vi "__uintDivide.vi"(8 "Base (decimal)":T1=10 items=["Binary"=2, "Octal"=8, "Decimal"=10, "Hexadecimal"=16, "Hexatrigesimal"=36, "ASCII"=64], 10 "Uint2 in":u8[](array[numeric]), 11 "Uint1 in":u8[](array[numeric])) -> (0 "Timing division":u32, 2 "floor(Uint1 / Uint1)":u8[](array[numeric]), 3 "Uint1 mod Uint2":u8[](array[numeric]))   [LabVIEW 2011, in "UintClass.lvclass"]
uses:
  UintClass.lvclass
  enumBase.ctl
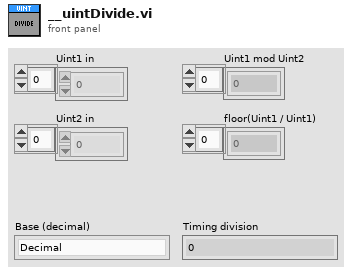
[diagram p1: front panel]
types:
  T1 = typedef "UintClass.lvclass/enumBase.ctl" = u16
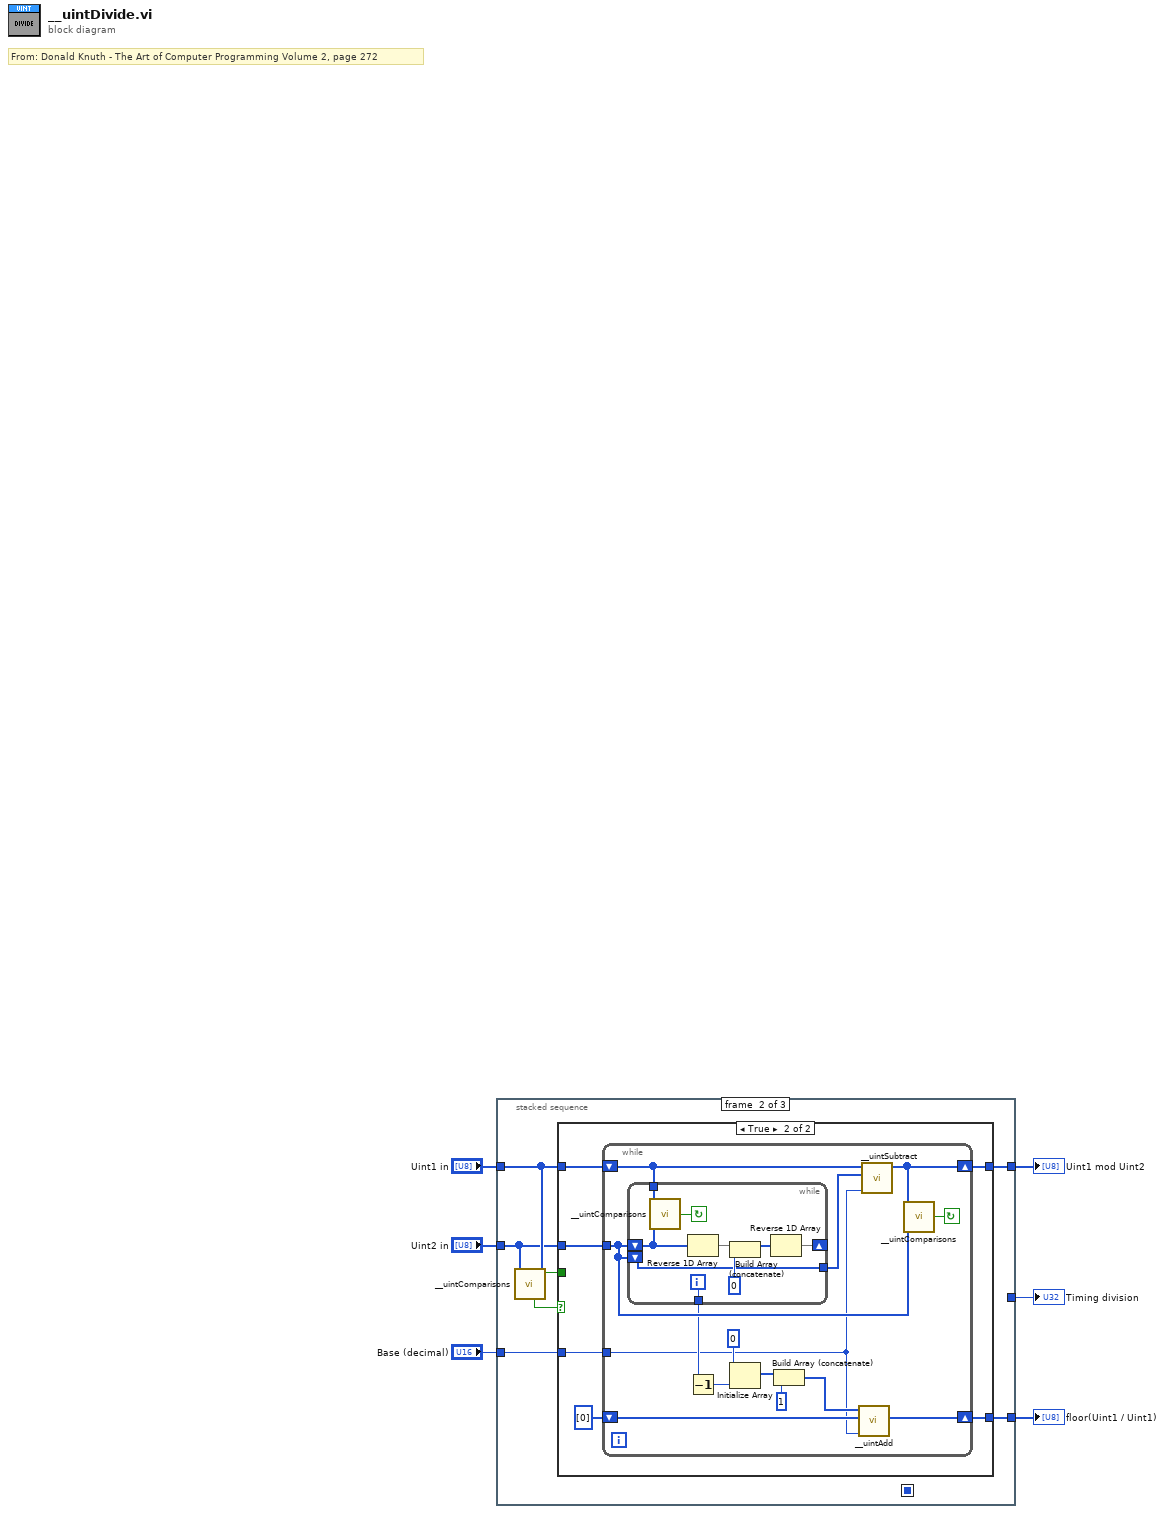
[diagram p0: block diagram]
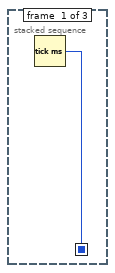
[diagram p2: hidden frame]
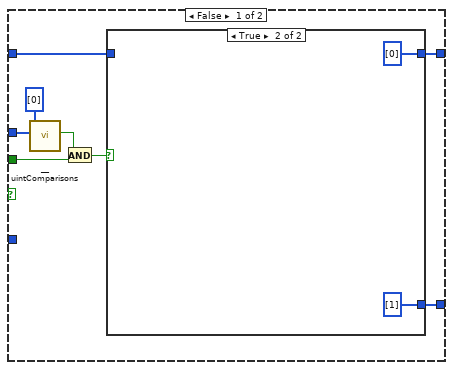
[diagram p3: hidden frame]
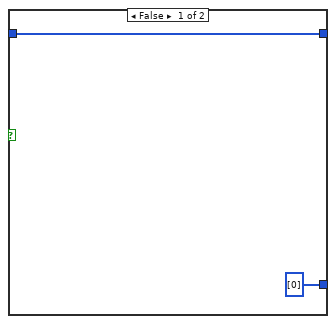
[diagram p4: hidden frame]
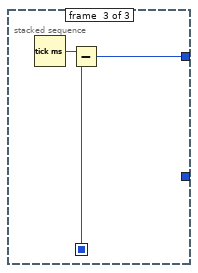
[diagram p5: hidden frame]
diagram:
  # "From: Donald Knuth - The Art of Computer Programming Volume 2, page 272"
  n1 = stacked-sequence {
    seq-local: [w7 _ _] -> [_ _ w57]
    tunnel: "Uint2 in" -> [_ w12 _]
    tunnel: "Uint1 in" -> [_ w13 _]
    tunnel: "Base (decimal)" -> [_ w14 _]
    tunnel: [_ w10 _] -> w4
    tunnel: [_ w11 _] -> w3
    tunnel: [_ _ w56] -> w1
    frame #0 {
      n2 = Tick Count (ms)() -> (millisecond timer value=w7:u32)
    }
    frame #1 {
      n3 = call "__uintComparisons.vi"("Uint2 in"=w12, "Uint1 in"=w13) -> ("Uint1 = Uint2"=w8:bool, "Uint1 > Uint2"=w9:bool)  [unwired: 3 in, 5 out]
      n4 = case shown="True" w9 {
        tunnel: w14 -> [_ w30]
        tunnel: w13 -> [w22 w32]
        tunnel: w12 -> [w19 w31]
        tunnel: [w21 w28] -> w11
        tunnel: [w20 w27] -> w10
        tunnel: w8 -> [w17 _]
        frame False {
          n5 = call "__uintComparisons.vi"("Uint2 in"=w19, "Uint1 in"=u8[] [0]) -> ("Uint1 != Uint2"=w15:bool)  [unwired: 3 in, 6 out]
          n6 = And(x=w15, y=w17) -> (x .and. y?=w16:bool)
          n7 = case shown="True" w16 {
            tunnel: w22 -> [w24 _]
            tunnel: [w24 u8[] [0] ("Uint2 in")] -> w21
            tunnel: [u8[] [0] ("Uint2 in") u8[] [1] ("Uint2 in")] -> w20
            frame False {
            }
            frame True {
            }
          }
        }
        frame True {
          n8 = while {
            tunnel: w31 -> [w44]
            tunnel: w30 -> [w34]
            shift-right: [w35] -> w28
            shift-left: w32 -> [w46]
            shift-right: [w36] -> w27
            shift-left: u8[] [0] ("Uint2 in") -> [w37]
            stop <- w33 continue-if-true
            n9 = while {
              tunnel: w46 -> [w55]
              shift-right: [w49] -> _
              shift-left: w44 -> [w53]
              shift-left: w44 -> [w48]
              tunnel: [w48] -> w45
              tunnel: [w47] -> w39
              i -> [w47]
              stop <- w54 continue-if-true
              n10 = call "__uintComparisons.vi"("Uint2 in"=w53, "Uint1 in"=w55) -> ("Uint1 >= Uint2"=w54:bool)  [unwired: 3 in, 6 out]
              n11 = Reverse 1D Array(array=w53) -> (reversed array=w52:u8[])
              n12 = Build Array (concatenate)(w52, u8 0 ("Numeric")) -> (w50:u8[])
              n13 = Reverse 1D Array(array=w50) -> (reversed array=w49:u8[])
            }
            n14 = Decrement(x=w39) -> (x-1=w43:i32)
            n15 = Initialize Array(u8 0 ("element"), w43) -> (w42:u8[])
            n16 = Build Array (concatenate)(w42, u8 1) -> (w38:u8[])
            n17 = call "__uintAdd.vi"("Base (decimal)"=w34, "Uint2 in"=w37, "Uint1 in"=w38) -> ("Uint1 + Uint2"=w36:u8[])  [unwired: 7 in, 1 out]
            n18 = call "__uintSubtract.vi"("Base (decimal)"=w34, "Uint2 in"=w45, "Uint1 in"=w46) -> ("Uint1 - Uint2"=w35:u8[])  [unwired: 7 in, 1 out]
            n19 = call "__uintComparisons.vi"("Uint2 in"=w44, "Uint1 in"=w35) -> ("Uint1 >= Uint2"=w33:bool)  [unwired: 3 in, 6 out]
          }
        }
      }
    }
    frame #2 {
      n20 = Tick Count (ms)() -> (millisecond timer value=w58:u32)
      n21 = Subtract(x=w58, y=w57) -> (x-y=w56:u32)
    }
  }
  "Timing division" <- w1
  "Uint1 mod Uint2" <- w3
  "floor(Uint1 / Uint1)" <- w4
